vi "DropTotes.vi"(11 "Boolean In":bool) -> (3 "Boolean Out":bool)   [LabVIEW 2014]
uses:
  Support Files/HandOffStates.ctl
  Support Files/Global Data!!!.vi
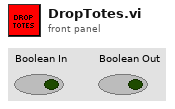
[diagram p1: front panel]
types:
  T1 = typedef "HandOffStates.ctl" = enum16{"Done", "Release2Stage", "Engage1Stage", "Raise1Stage", "Pause"}
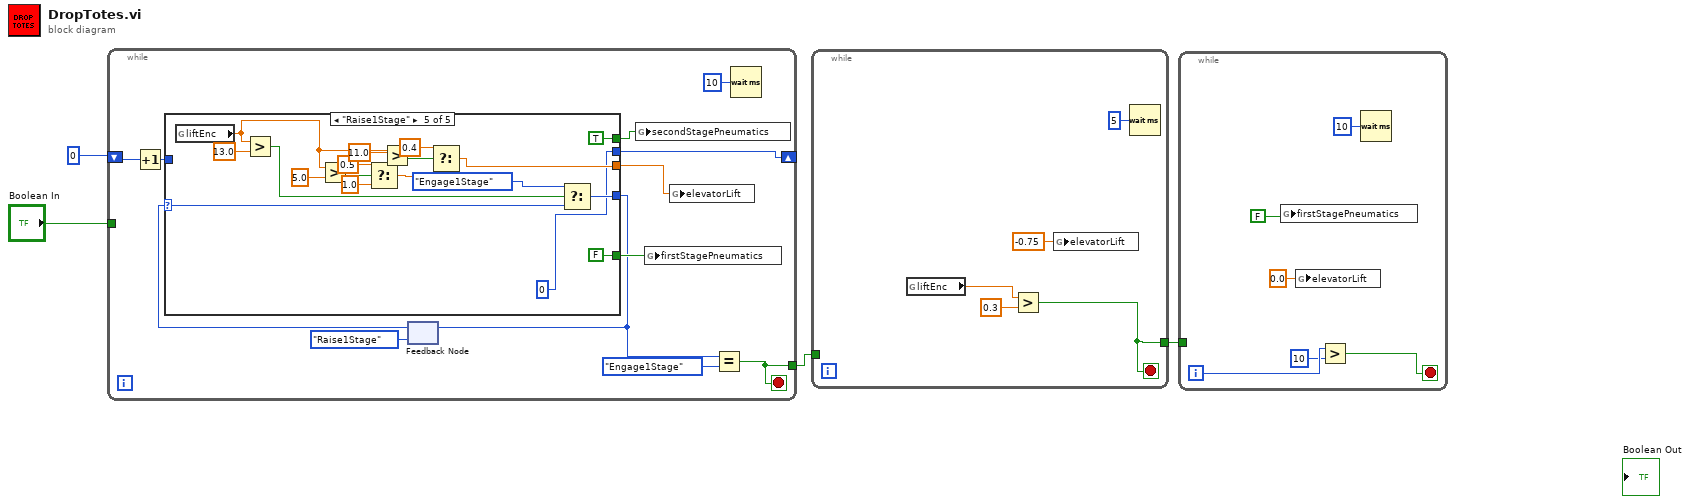
[diagram p0: block diagram]
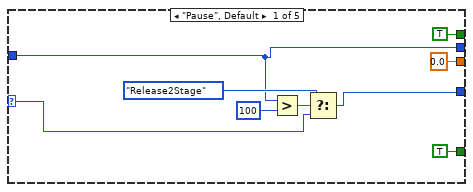
[diagram p2: hidden frame]
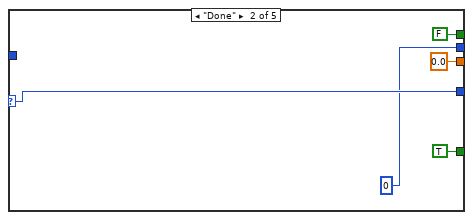
[diagram p3: hidden frame]
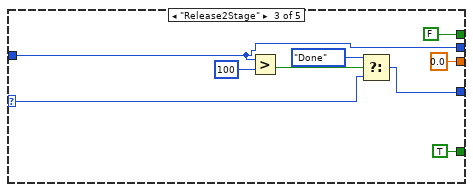
[diagram p4: hidden frame]
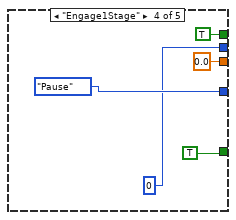
[diagram p5: hidden frame]
diagram:
  n1 = while {
    tunnel: "Boolean In" -> [_]
    tunnel: [w9] -> w3
    shift-right: [w5] -> _
    shift-left: 0 -> [w7]
    stop <- w9 stop-if-true
    n2 = Increment(x=w7) -> (x+1=w6:i32)
    n3 = feedback #1(HandOffStates."Raise1Stage") -> (w15:T1)
    n4 = case shown="\"Raise1Stage\"" w15 {
      selector: w15 -> [w22 w28 w36 _ w62]
      tunnel: [w23 w28 w35 HandOffStates."Pause" ("t") w61] -> w11
      tunnel: [0.0 ("f") 0.0 ("f") 0.0 ("f") 0.0 ("f") w48] -> w16
      tunnel: [TRUE TRUE TRUE TRUE FALSE] -> w13
      tunnel: [TRUE FALSE FALSE TRUE TRUE] -> w14
      tunnel: w6 -> [w17 _ w31 _ _]
      tunnel: [w17 0 ("Numeric") w31 0 ("Numeric") 0 ("Numeric")] -> w5
      frame "Pause", Default {
        n5 = Greater?(x=w17, y=100) -> (0:w24:bool)
        n6 = Select(t=HandOffStates."Release2Stage", s=w24, f=w22) -> (s? t:f=w23:T1)
      }
      frame "Done" {
      }
      frame "Release2Stage" {
        n7 = Greater?(x=w31, y=100) -> (0:w37:bool)
        n8 = Select(t=HandOffStates."Done", s=w37, f=w36) -> (s? t:f=w35:T1)
      }
      frame "Engage1Stage" {
      }
      frame "Raise1Stage" {
        n9 = global read "Global Data!!!.vi" "liftEnc"() -> (w50:dbl)
        n10 = Greater?(x=w50, y=13.0) -> (0:w59:bool)
        n11 = Greater?(x=w50, y=5.0) -> (0:w56:bool)
        n12 = Select(t=0.5, s=w56, f=1.0) -> (s? t:f=w51:dbl)
        n13 = Greater?(x=w50, y=11.0) -> (0:w52:bool)
        n14 = Select(t=0.4, s=w52, f=w51) -> (s? t:f=w48:dbl)
        n15 = Select(t=HandOffStates."Engage1Stage", s=w59, f=w62) -> (s? t:f=w61:T1)
      }
    }
    n16 = feedback-in #1(w11) -> ()
    n17 = global write "Global Data!!!.vi" "secondStagePneumatics"(w14) -> ()
    n18 = global write "Global Data!!!.vi" "firstStagePneumatics"(w13) -> ()
    n19 = global write "Global Data!!!.vi" "elevatorLift"(w16) -> ()
    n20 = Equal?(x=w11, y=HandOffStates."Engage1Stage") -> (x = y?=w9:bool)
    n21 = Wait (ms)(milliseconds to wait=u32 10) -> ()  [unwired: 1 out]
  }
  n22 = while {
    tunnel: w3 -> [_]
    tunnel: [w64] -> w2
    stop <- w64 stop-if-true
    n23 = global read "Global Data!!!.vi" "liftEnc"() -> (w66:dbl)
    n24 = Greater?(x=w66, y=0.3) -> (0:w64:bool)
    n25 = global write "Global Data!!!.vi" "elevatorLift"(-0.75 ("elevatorLift")) -> ()
    n26 = Wait (ms)(milliseconds to wait=u32 5) -> ()  [unwired: 1 out]
  }
  n27 = while {
    tunnel: w2 -> [_]
    i -> [w71]
    stop <- w68 stop-if-true
    n28 = global write "Global Data!!!.vi" "firstStagePneumatics"(FALSE ("firstStagePneumatics")) -> ()
    n29 = global write "Global Data!!!.vi" "elevatorLift"(0.0 ("elevatorLift")) -> ()
    n30 = Greater?(x=w71, y=10) -> (0:w68:bool)
    n31 = Wait (ms)(milliseconds to wait=u32 10) -> ()  [unwired: 1 out]
  }
